vi "Test_Copy_Image_No_Mask_Greyscale.vi"(8 "error in (no error)":errorcluster, 11 "Test Case In":refnum<class "Image.lvclass">) -> (0 "error out":errorcluster, 3 "Test Case Out":refnum<class "Image.lvclass">)   [LabVIEW 2020, in "g_ar_toolkit.test.lvlib" / "Image.lvclass"]
uses:
  Image.lvclass
  Image.lvclass/Image.ctl
  g_ar_toolkit.image/g_ar_toolkit.image.lvlib
  g_ar_toolkit.image/Image Size (Fixed).ctl
  g_ar_toolkit.image/CreateEmptyImageGreyscale.vi
  g_ar_toolkit.image/CopyImageNoMaskGreyscale.vi
  4993e8ee-a06a-463a-9684-69129f64d5ce.vi
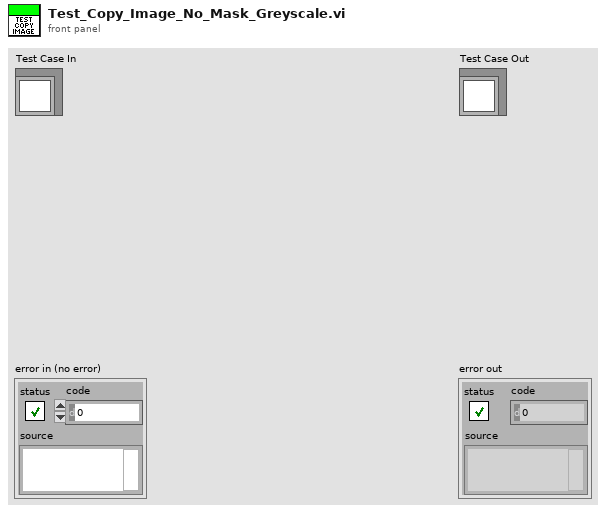
[diagram p1: front panel]
types:
  T1 = typedef "g_ar_toolkit.image.lvlib/Image Size (Fixed).ctl" = cluster{"Width":u16, "Height":u16}
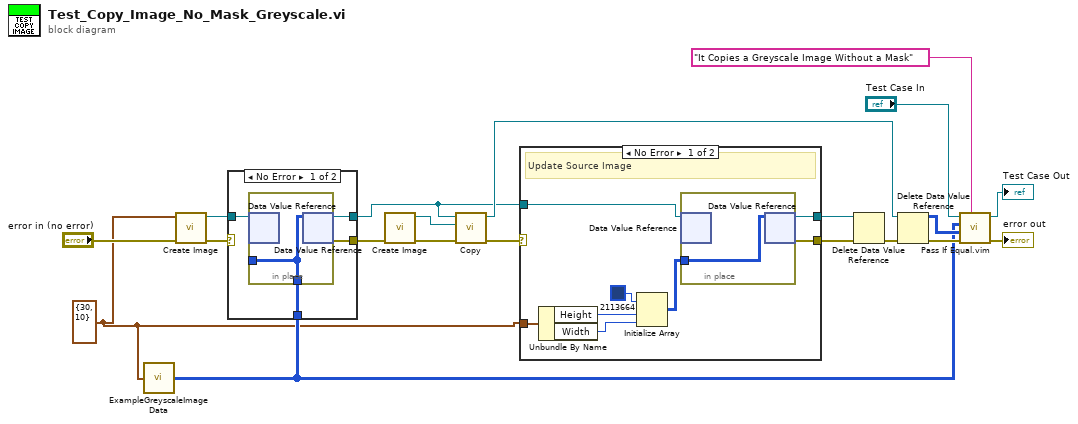
[diagram p0: block diagram]
diagram:
  w1 = T1 {"Width"=30, "Height"=10} ("Preallocated Image Size (Default - 0,0)")
  n1 = call "ExampleGreyscaleImageData.vi"("Image Size"=w1) -> ("GreyscaleImage"=w4:u8[][])
  n2 = call-poly "Create Image.vi"("error in (no error)"="error in (no error)", "Preallocated Image Size (Default 0,0)"=w1) -> ("error out"=w14:errorcluster, "New Greyscale Image"=w15:refnum<data-value>)  [unwired: 8 in]
  n3 = case shown="No Error" w14 {
    selector: w14 -> [_ w26]
    tunnel: w15 -> [w24 w27]
    tunnel: [w23 w27] -> w3
    tunnel: [w22 w26] -> w13
    tunnel: w4 -> [w21 _]
    frame No Error {
      n4 = in-place {
        in-place-border: [w25] -> _
        in-place-border: w21 -> [w25]
        n5 = in-place-dvr #1(w24) -> ()  [unwired: 2 out]
        n6 = in-place-dvr #1(w25) -> (w23:refnum<data-value>, w22:errorcluster)
      }
    }
    frame Error {
    }
  }
  n7 = call-poly "Create Image.vi"("error in (no error)"=w13) -> ("error out"=w12:errorcluster, "New Greyscale Image"=w2:refnum<data-value>)  [unwired: 9 in]
  n8 = call-poly "Copy.vi"("error in (no error)"=w12, "Greyscale Image Destination"=w2, "Greyscale Image Source"=w3) -> ("error out"=w9:errorcluster, "Greyscale Image Destination (duplicate)"=w6:refnum<data-value>)  [unwired: 7 in]
  n9 = case shown="No Error" w9 {
    selector: w9 -> [_ w37]
    tunnel: w3 -> [w35 w38]
    tunnel: [w34 w38] -> w7
    tunnel: [w33 w37] -> w8
    tunnel: w1 -> [w30 _]
    frame No Error {
      # "Update Source Image"
      n10 = Unbundle By Name(w30) -> ("Height"=w32:u16, "Width"=w31:u16)
      n11 = Initialize Array(u32 2113664, w32, w31) -> (w28:u32[][])
      n12 = in-place {
        in-place-border: w28 -> [w36]
        n13 = in-place-dvr #2(w35) -> ()  [unwired: 2 out]
        n14 = in-place-dvr #2(w36) -> (w34:refnum<data-value>, w33:errorcluster)
      }
    }
    frame Error {
    }
  }
  n15 = Delete Data Value Reference(data value reference=w7, error in=w8) -> (error out=w11:errorcluster)  [unwired: 1 out]
  n16 = Delete Data Value Reference(data value reference=w6, error in=w11) -> (data value=w5:u8[][], error out=w10:errorcluster)
  n17 = call "Pass If Equal.vim"("Description"="It Copies a Greyscale Image Without a Mask", "error in (no error)"=w10, "Actual"=w5, "Expected"=w4, "LUnit Test Case In"="Test Case In") -> ("error out"=→"error out":errorcluster, "LUnit Test Case Out"=→"Test Case Out":refnum<class "Image.lvclass">)  [unwired: 5 in]
